vi "final project.vi"() -> ()   [LabVIEW 2016]
panel:
  out "Array":T1(array[cluster])
  in  "color(black) 2":u32(colorbox)
  in  "color(black)":u32(colorbox)
  in  "Send Button":bool
  in  "DAC2":dbl
  in  "DAC1":dbl
  out "Y":dbl
  out "X":dbl
  in  "stop":bool
  in  "Display History":bool
  out "2D Picture":picture
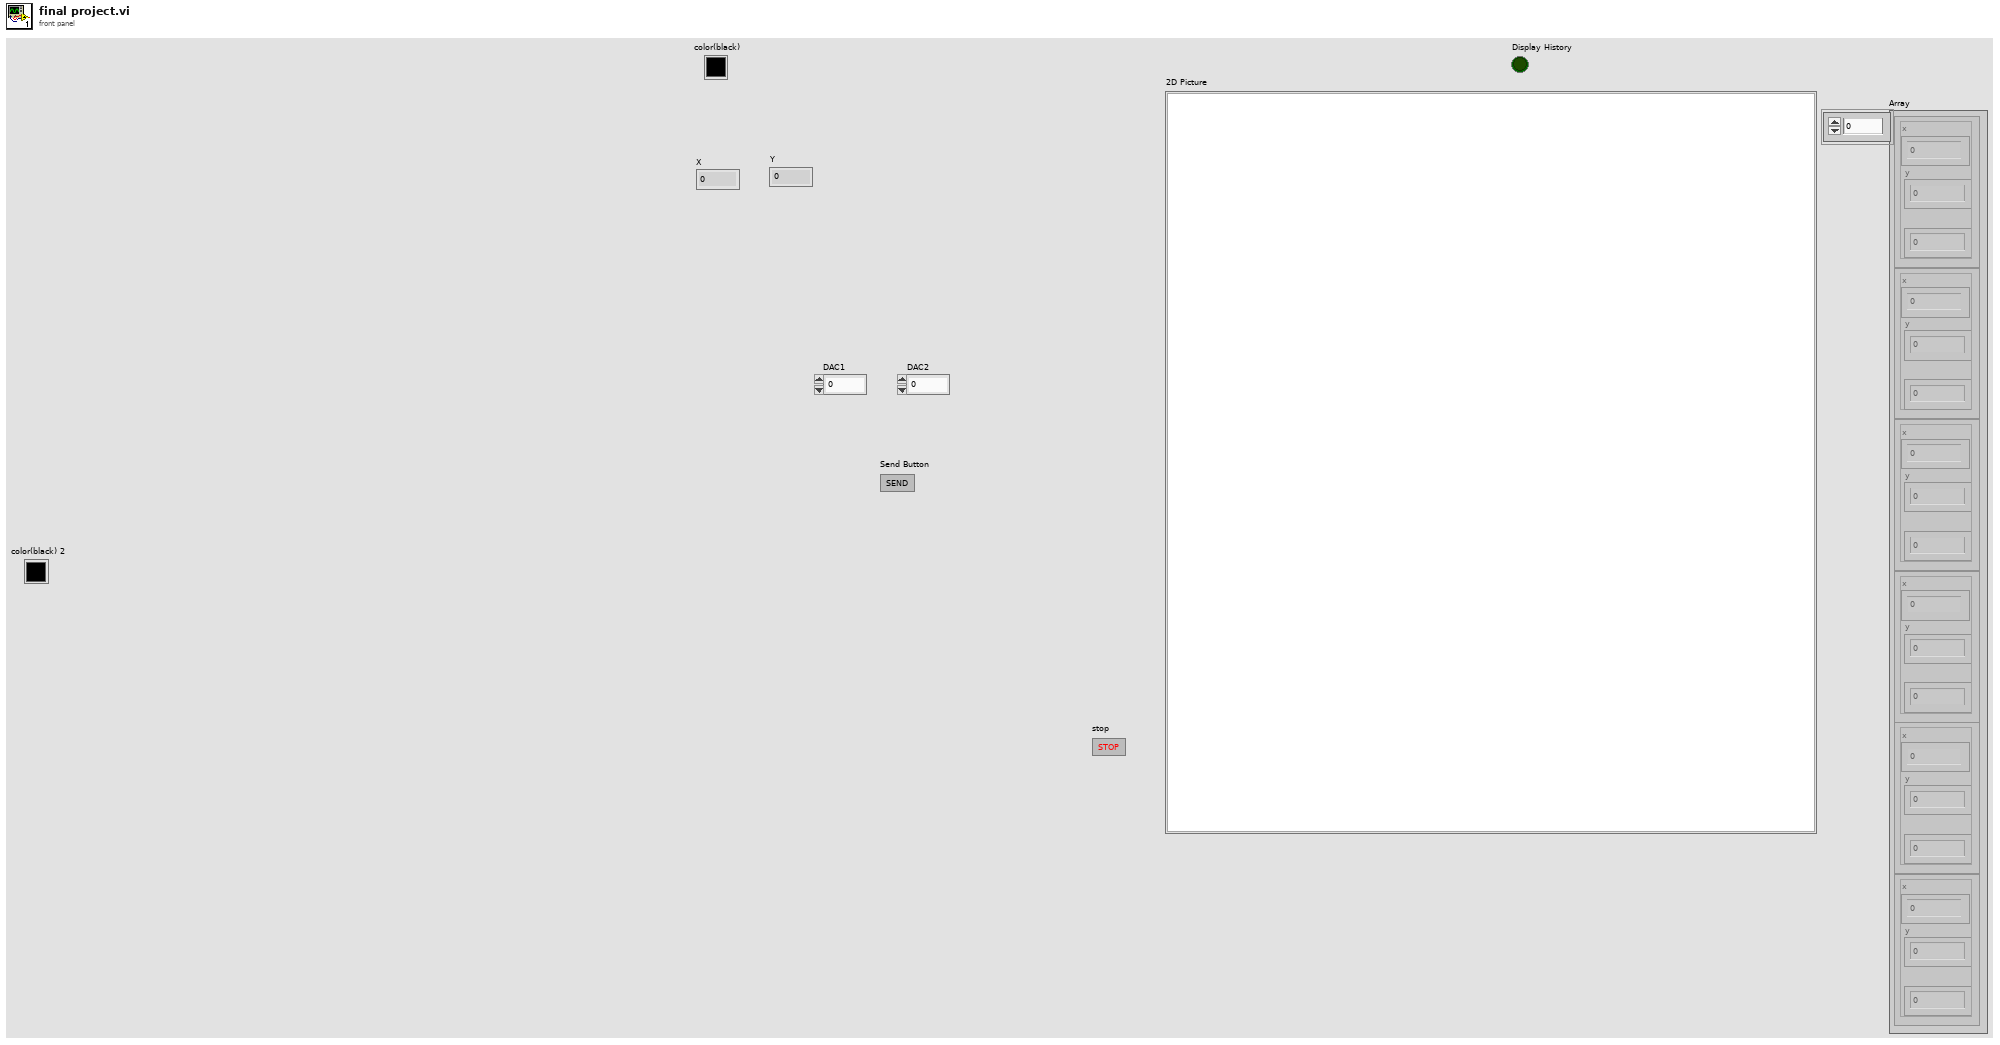
[diagram p1: front panel]
types:
  T1 = cluster{"x":dbl, "y":dbl, "Numeric Control":i16}[]
  T2 = cluster{"Width":u16, "Style":enum32{"Solid", "Dash", "Dot", "DashDot", "DashDotDot"}}
  T3 = enum16{"Standard", "Buffered", "CRLF", "Immediate"}
  T4 = cluster{"default value 5":dbl, "default value 6":dbl, "default value 7":i32}
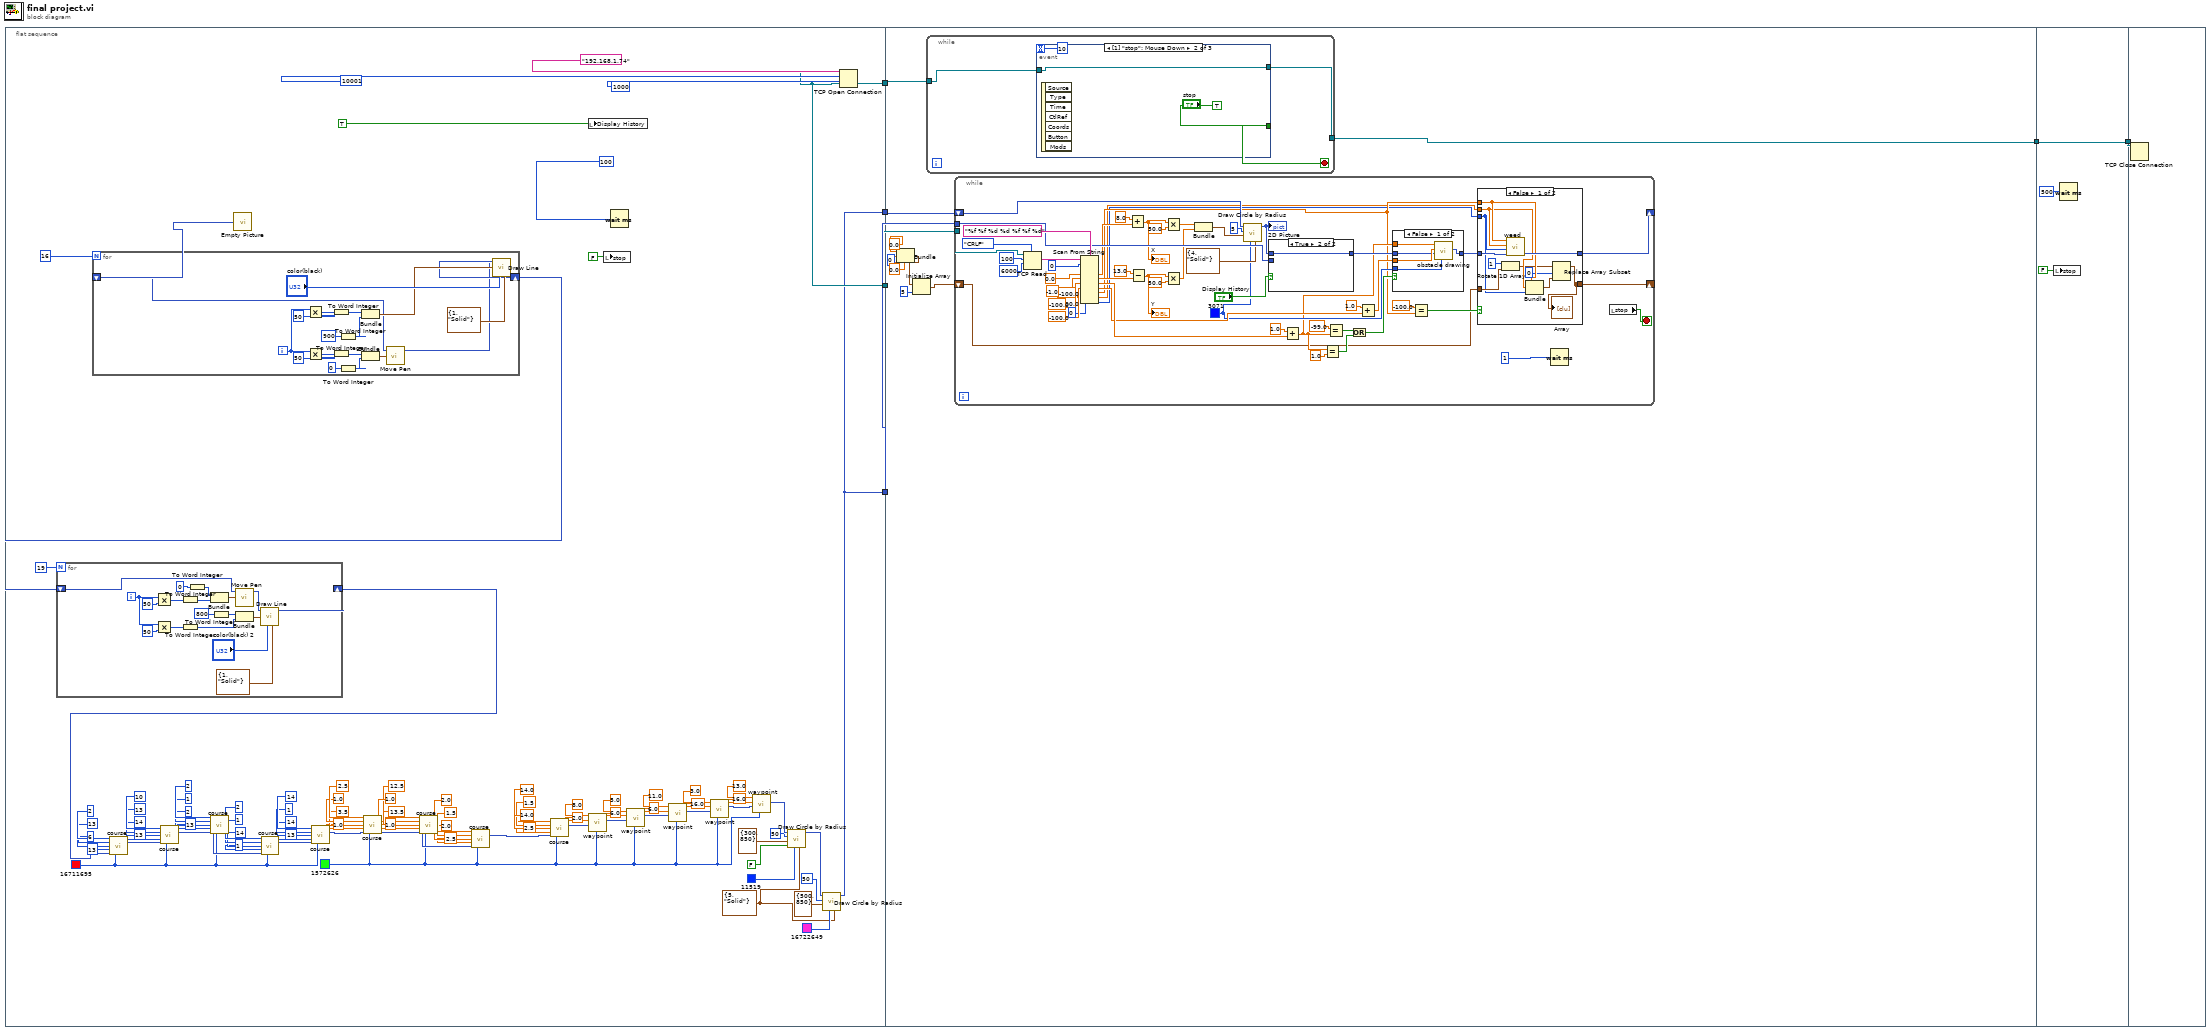
[diagram p0: block diagram]
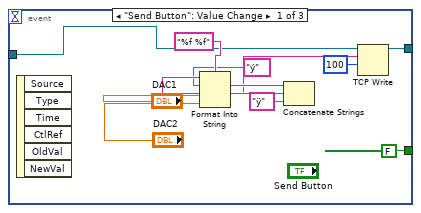
[diagram p5: hidden frame]
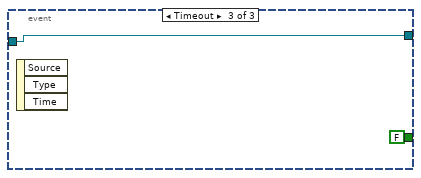
[diagram p6: hidden frame]
diagram:
  n1 = flat-sequence {
    tunnel: [w86] -> w6
    tunnel: [w86] -> w5
    tunnel: [w29] -> w2
    tunnel: [w29] -> w1
    tunnel: w6 -> [w135]
    tunnel: w5 -> [w134]
    tunnel: [w137] -> w4
    tunnel: w2 -> [w136]
    tunnel: w1 -> [w133]
    tunnel: w4 -> [w235]
    tunnel: [w235] -> w3
    tunnel: w3 -> [w236]
    frame #0 {
      w30 = T2 {"Width"=5, "Style"=enum."Solid"} ("pen")
      w7 = u32 1572626 ("color(black)")
      w54 = u32 16711695 ("color(black)")
      n2 = call "Empty Picture"() -> ("empty picture"=w82:picture)
      n3 = for {
        N: 16 -> [_]
        shift-right: [w118] -> w81
        shift-left: w82 -> [w117]
        i -> [w113]
        n4 = Multiply(x=w113, y=50) -> (x*y=w124:i32)
        n5 = Multiply(x=w113, y=50) -> (x*y=w116:i32)
        n6 = To Word Integer(number=w124) -> (16bit integer=w123:i16)
        n7 = To Word Integer(number=w116) -> (16bit integer=w114:i16)
        n8 = To Word Integer(number=900) -> (16bit integer=w120:i16)
        n9 = To Word Integer(number=0) -> (16bit integer=w111:i16)
        n10 = Bundle(w123, w120) -> (w122:cluster{i16, i16})  [unwired: 1 in]
        n11 = Bundle(w114, w111) -> (w110:cluster{i16, i16})  [unwired: 1 in]
        n12 = call <vilib>:"Move Pen.vi"("new position"=w110, "picture"=w117) -> ("new picture"=w109:picture)  [unwired: 3 in]
        n13 = call <vilib>:"Draw Line.vi"("picture"=w109, "end point"=w122, "color(black)"="color(black)", "pen"=T2 {"Width"=1, "Style"=enum."Solid"}) -> ("new picture"=w118:picture)  [unwired: 5 in]
      }
      n14 = for {
        N: 19 -> [_]
        shift-right: [w102] -> w79
        shift-left: w81 -> [w101]
        i -> [w98]
        n15 = Multiply(x=w98, y=50) -> (x*y=w100:i32)
        n16 = Multiply(x=w98, y=50) -> (x*y=w106:i32)
        n17 = To Word Integer(number=w100) -> (16bit integer=w93:i16)
        n18 = To Word Integer(number=w106) -> (16bit integer=w92:i16)
        n19 = To Word Integer(number=0) -> (16bit integer=w94:i16)
        n20 = Bundle(w94, w93) -> (w96:cluster{i16, i16})  [unwired: 1 in]
        n21 = To Word Integer(number=800) -> (16bit integer=w91:i16)
        n22 = call <vilib>:"Move Pen.vi"("new position"=w96, "picture"=w101) -> ("new picture"=w95:picture)  [unwired: 3 in]
        n23 = Bundle(w91, w92) -> (w105:cluster{i16, i16})  [unwired: 1 in]
        n24 = call <vilib>:"Draw Line.vi"("picture"=w95, "end point"=w105, "color(black)"="color(black) 2", "pen"=T2 {"Width"=1, "Style"=enum."Solid"}) -> ("new picture"=w102:picture)  [unwired: 5 in]
      }
      n25 = call "course.vi"("x1"=2, "y 1"=13, "x2"=6, "y 2"=13, "picture"=w79, "color(black)"=w54) -> ("new picture"=w74:picture)  [unwired: 9 in]
      n26 = call "course.vi"("x1"=10, "y 1"=13, "x2"=14, "y 2"=13, "picture"=w74, "color(black)"=w54) -> ("new picture"=w73:picture)  [unwired: 9 in]
      n27 = call "course.vi"("x1"=2, "y 1"=1, "x2"=2, "y 2"=13, "picture"=w73, "color(black)"=w54) -> ("new picture"=w72:picture)  [unwired: 9 in]
      n28 = call "course.vi"("x1"=2, "y 1"=1, "x2"=14, "y 2"=1, "picture"=w72, "color(black)"=w54) -> ("new picture"=w71:picture)  [unwired: 9 in]
      n29 = call "course.vi"("x1"=14, "y 1"=1, "x2"=14, "y 2"=13, "picture"=w71, "color(black)"=w54) -> ("new picture"=w9:picture)  [unwired: 9 in]
      n30 = call "course.vi"("x1"=2.5, "y 1"=1.0, "x2"=3.5, "y 2"=1.0, "picture"=w9, "color(black)"=w7) -> ("new picture"=w12:picture)  [unwired: 9 in]
      n31 = call "course.vi"("x1"=12.5, "y 1"=1.0, "x2"=13.5, "y 2"=1.0, "picture"=w12, "color(black)"=w7) -> ("new picture"=w11:picture)  [unwired: 9 in]
      n32 = call "course.vi"("x1"=2.0, "y 1"=1.5, "x2"=2.0, "y 2"=2.5, "picture"=w11, "color(black)"=w7) -> ("new picture"=w10:picture)  [unwired: 9 in]
      n33 = call "course.vi"("x1"=14.0, "y 1"=1.5, "x2"=14.0, "y 2"=2.5, "picture"=w10, "color(black)"=w7) -> ("new picture"=w8:picture)  [unwired: 9 in]
      n34 = local write "Display History"(TRUE ("Display History")) -> ()
      n35 = call "waypoint.vi"("color(black)"=w7, "picture"=w8, "waypointy"=2.0, "waypointx"=8.0) -> ("new picture"=w53:picture)  [unwired: 7 in]
      n36 = local write "stop"(FALSE ("stop")) -> ()
      n37 = Wait (ms)(milliseconds to wait=u32 100) -> ()  [unwired: 1 out]
      n38 = call "waypoint.vi"("color(black)"=w7, "picture"=w53, "waypointy"=6.0, "waypointx"=5.0) -> ("new picture"=w52:picture)  [unwired: 7 in]
      n39 = call "waypoint.vi"("color(black)"=w7, "picture"=w52, "waypointy"=6.0, "waypointx"=11.0) -> ("new picture"=w51:picture)  [unwired: 7 in]
      n40 = call "waypoint.vi"("color(black)"=w7, "picture"=w51, "waypointy"=16.0, "waypointx"=3.0) -> ("new picture"=w50:picture)  [unwired: 7 in]
      n41 = call "waypoint.vi"("color(black)"=w7, "picture"=w50, "waypointy"=16.0, "waypointx"=13.0) -> ("new picture"=w39:picture)  [unwired: 7 in]
      n42 = call <vilib>:"Draw Circle by Radius.vi"("pen"=w30, "color(black)"=u32 11519, "fill?(F)"=FALSE, "pixel center"=cluster{"horizontal":i16, "vertical":i16} {"horizontal"=300, "vertical"=850}, "radius"=i16 50, "picture"=w39) -> ("new picture"=w34:picture)  [unwired: 5 in]
      n43 = call <vilib>:"Draw Circle by Radius.vi"("pen"=w30, "color(black)"=u32 16722649, "pixel center"=cluster{"horizontal":i16, "vertical":i16} {"horizontal"=500, "vertical"=850}, "radius"=i16 50, "picture"=w34) -> ("new picture"=w29:picture)  [unwired: 6 in]
      n44 = TCP Open Connection(address="192.168.1.74", remote port or service name=u16 10001, timeout ms (60000)=1000) -> (connection ID=w86:refnum<k5>)  [unwired: 2 in, 1 out]
    }
    frame #1 {
      n45 = Bundle("x"=0.0, "x"=0.0, i16 0) -> (w130:cluster{"x":dbl, "x":dbl, i16})  [unwired: 1 in]
      n46 = Initialize Array(w130, 5 ("dimension size")) -> (w132:cluster{"x":dbl, "x":dbl, i16}[])
      n47 = while {
        tunnel: [w215] -> w137
        tunnel: w135 -> [w214]
        stop <- w216 stop-if-true
        n48 = event shown="[1] \"stop\": Mouse Down" {
          selector: _ -> [_ _ _]
          dyn-events: _ -> [_ _ _]
          timeout: 10 -> [_ _ _]
          tunnel: [FALSE TRUE ("stop") FALSE] -> w216
          tunnel: [w219 w229 w232] -> w215
          tunnel: w214 -> [w218 w229 w232]
          event "Send Button": Value Change {
            n49 = event-data() -> ()  [unwired: 1 in, 6 out]
            n50 = Format Into String(format string="%f %f", "DAC1", "DAC2") -> (resulting string=w224:string)  [unwired: 2 in, 1 out]
            n51 = Concatenate Strings("ý" ("string"), w224, "ÿ" ("string")) -> (w221:string)
            n52 = TCP Write(connection ID=w218, data in=w221, 9:100 ("timeout ms (25000)")) -> (connection ID out=w219:refnum<k5>)  [unwired: 1 in, 2 out]
          }
          event "stop": Mouse Down {
            n53 = event-data() -> ()  [unwired: 1 in, 7 out]
          }
          event Timeout {
            n54 = event-data() -> ()  [unwired: 1 in, 3 out]
          }
        }
      }
      n55 = while {
        shift-right: [w143] -> _
        shift-left: w136 -> [w179]
        tunnel: w134 -> [w178]
        tunnel: w133 -> [w177]
        shift-right: [w138] -> _
        shift-left: w132 -> [w139]
        stop <- w180 stop-if-true
        w157 = u32 3071
        n56 = TCP Read(connection ID=w178, bytes to read=100, 7:T3."CRLF" ("mode (standard)"), 9:6000 ("timeout ms (25000)")) -> (data out=w188:string)  [unwired: 1 in, 2 out]
        n57 = Scan From String(format string="%f %f %d %d %f %f %d", input string=w188, initial scan location=u32 0, default 1=0.0 ("default value 1"), default 2=-1.0 ("default value 2"), default 3=-100.0 ("default value 3"), default 4=-100.0 ("default value 4"), default 5=-100.0 ("default value 5"), default 6=-100.0 ("default value 6"), default 7=0 ("default value 7")) -> (output 1=w168:dbl, output 2=w156:dbl, output 3=w164:dbl, output 4=w161:dbl, output 5=w147:dbl, output 6=w146:dbl, output 7=w145:i32)  [unwired: 1 in, 3 out]
        n58 = Add(x=8.0, y=w168) -> (x+y=w166:dbl)
        "X" <- w166
        n59 = Subtract(x=13.0 ("y"), y=w156) -> (x-y=w165:dbl)
        "Y" <- w165
        n60 = Multiply(x=w166, y=50.0) -> (x*y=w169:dbl)
        n61 = Multiply(x=w165, y=50.0) -> (x*y=w170:dbl)
        n62 = Bundle(w169, w170) -> (w174:cluster{dbl, dbl})  [unwired: 1 in]
        n63 = call <vilib>:"Draw Circle by Radius.vi"("pen"=T2 {"Width"=4, "Style"=enum."Solid"}, "color(black)"=w157, "pixel center"=w174, "radius"=i16 5, "picture"=w179) -> ("new picture"=w171:picture)  [unwired: 6 in]
        "2D Picture" <- w171
        n64 = case shown="True" "Display History" {
          tunnel: [w212 w213] -> w159
          tunnel: w177 -> [w212 _]
          tunnel: w171 -> [_ w213]
          frame False {
          }
          frame True {
          }
        }
        n65 = Add(x=1.0, y=w164) -> (x+y=w153:dbl)
        n66 = Equal?(x=w153, y=1.0) -> (x = y?=w151:bool)
        n67 = Equal?(x=-99.0, y=w153) -> (x = y?=w154:bool)
        n68 = Or(x=w154, y=w151) -> (x .or. y?=w150:bool)
        n69 = Add(x=1.0, y=w161) -> (x+y=w158:dbl)
        n70 = case shown="False" w150 {
          tunnel: w159 -> [w208 w211]
          tunnel: w153 -> [w210 _]
          tunnel: w158 -> [w209 _]
          tunnel: [w207 w211] -> w144
          tunnel: w157 -> [w206 _]
          frame False {
            n71 = call "obstacle drawing.vi"("color(black)"=w206, "picture"=w208, "Col input"=w209, "Row input"=w210) -> ("new picture"=w207:picture)  [unwired: 7 in]
          }
          frame True {
          }
        }
        n72 = Equal?(x=-100.0, y=w147) -> (x = y?=w148:bool)
        n73 = case shown="False" w148 {
          tunnel: w147 -> [w201 _]
          tunnel: w146 -> [w200 _]
          tunnel: w145 -> [w194 _]
          tunnel: w144 -> [w203 w205]
          tunnel: [w202 w205] -> w143
          tunnel: [w193 w204] -> w138
          tunnel: w139 -> [w197 w204]
          frame False {
            n74 = Rotate 1D Array(1:w197, 2:1 ("n")) -> (0:w196:cluster{"x":dbl, "x":dbl, i16}[])
            n75 = call "weed.vi"("picture"=w203, "color"=w194, "y"=w200, "x"=w201) -> ("new picture"=w202:picture)  [unwired: 7 in]
            n76 = Bundle("default value 5"=w201, "default value 6"=w200, "default value 7"=w194) -> (w199:T4)  [unwired: 1 in]
            n77 = Replace Array Subset(array=w196, new element=w199, index=0) -> (w193:cluster{"x":dbl, "x":dbl, i16}[])
            "Array" <- w193
          }
          frame True {
          }
        }
        n78 = Wait (ms)(milliseconds to wait=u32 1) -> ()  [unwired: 1 out]
        n79 = local read "stop"() -> (w180:bool)
      }
    }
    frame #2 {
      n80 = local write "stop"(FALSE ("stop")) -> ()
      n81 = Wait (ms)(milliseconds to wait=u32 500) -> ()  [unwired: 1 out]
    }
    frame #3 {
      n82 = TCP Close Connection(connection ID=w236) -> ()  [unwired: 2 in, 2 out]
    }
  }
